vi "Read Module Model (Module EEPROM).vi"(8 "error in":errorcluster, 11 "Refnum in":refnum<k20>) -> (0 "error out":errorcluster, 2 "Module Model":string, 3 "Refnum out":refnum<k20>)   [LabVIEW 2016, in "SMI.lvlib" / "C Series Module.lvclass"]
uses:
  C Series Module.lvclass
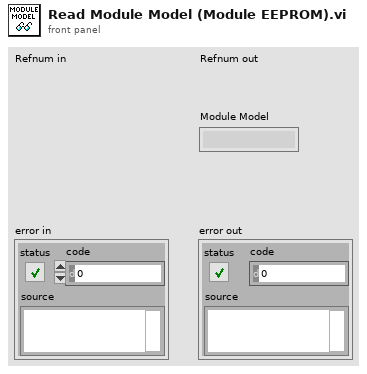
[diagram p1: front panel]
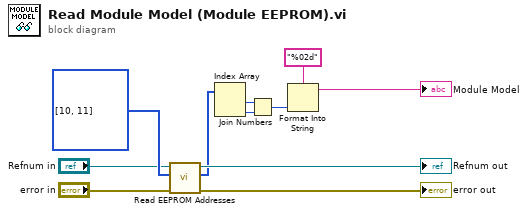
[diagram p0: block diagram]
diagram:
  n1 = call "Read EEPROM Addresses.vi"("error in (no error)"="error in", "Addresses"=u16[] [10, 11], "Refnum in"="Refnum in") -> ("error out"=→"error out":errorcluster, "Data"=w5:u8[], "Refnum out"=→"Refnum out":refnum<k20>)  [unwired: 6 in]
  n2 = Index Array(array=w5) -> (element #1=w3:u8, element #2=w4:u8)  [unwired: 2 in]
  n3 = Join Numbers(hi=w3, lo=w4) -> ((hi.lo)=w2:u16)
  n4 = Format Into String(format string="%02d", w2) -> (resulting string=→"Module Model":string)  [unwired: 2 in, 1 out]
